vi "variant2Attributes.vi"(0 "HGV_PVBase":refnum<class "HGF_DSCSubscriber.lvclass">, 2 "rawData":variant, 3 "typeDescriptor":string, 5 "error in (no error)":errorcluster) -> (14 "HGV_PVBase":refnum<class "HGF_DSCSubscriber.lvclass">, 15 "no link":bool, 16 "Parameter":variant, 17 "typeDescriptor":string, 19 "error out":errorcluster)   [LabVIEW 2012, in "HGF_DSC.lvlib" / "HGF_DSCSubscriber.lvclass"]
doc: "Convert raw data value of variant to variant attributes Pn, n=0,1,2,..."
uses:
  HGF_DSCSubscriber.lvclass
  HGF_SV/HGF_SVSubscriber/HGF_SVSubscriber.lvclass
  HGF_DSCSubscriber.lvclass/HGF_DSCSubscriber.ctl
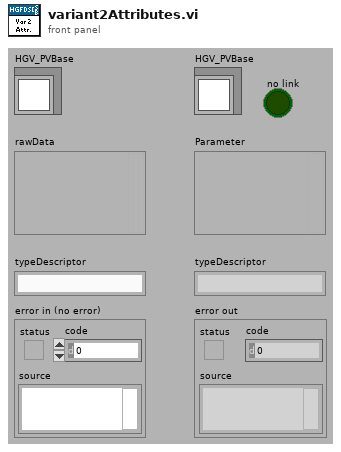
[diagram p1: front panel]
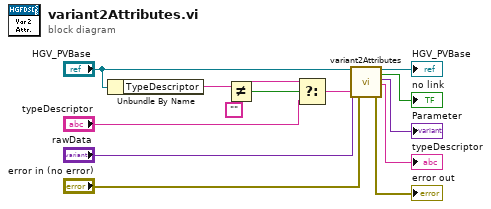
[diagram p0: block diagram]
diagram:
  n1 = Unbundle By Name("HGV_PVBase") -> ("TypeDescriptor"=w3:string)
  n2 = Not Equal?(x=w3, y="") -> (x != y?=w4:bool)
  n3 = Select(t=w3, s=w4, f="typeDescriptor") -> (s? t:f=w1:string)
  n4 = call-parent "variant2Attributes.vi"("HGV_PVBase"="HGV_PVBase", "rawData"="rawData", "typeDescriptor"=w1, "error in (no error)"="error in (no error)") -> ("HGV_PVBase"=→"HGV_PVBase":refnum<class "HGF_DSCSubscriber.lvclass">, "no link"=→"no link":bool, "Parameter"=→"Parameter":variant, "typeDescriptor"=→"typeDescriptor":string, "error out"=→"error out":errorcluster)  [unwired: 11 out]
